vi "LaunchEditor.vi"(8 "error in (no error)":errorcluster {"code" format="Error %.0f"}, 10 "Editor Events":T1, 11 "Parser Settings In":refnum<class "Parser Settings.lvclass">) -> (0 "error out":errorcluster {"code" format="Error %.0f"}, 2 "VI Refnum":refnum<vi>, 3 "Parser Settings Out":refnum<class "Parser Settings.lvclass">)   [LabVIEW 2023, in "VIDoc Parsing.lvlib" / "Parser Settings.lvclass"]
uses:
  Parser Settings.lvclass
  Editors/VIDoc Editor/Editor Events Cluster.ctl
  Editor.vi
  Parser Settings.lvclass/Parser Settings.ctl
  Editors/VIDoc Editor/VIDocEditor.lvclass
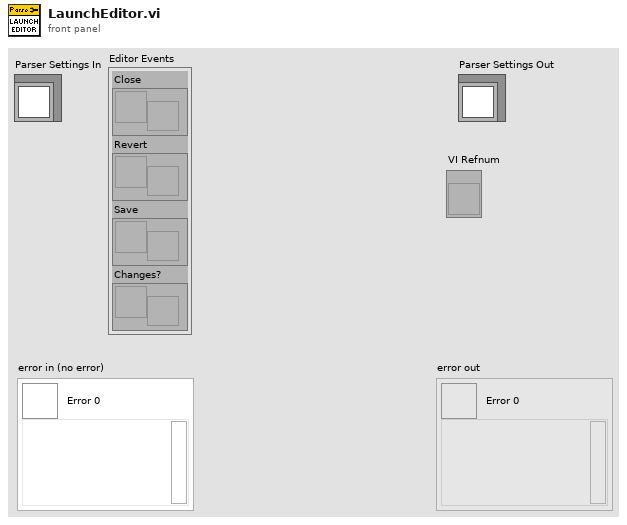
[diagram p1: front panel]
types:
  T1 = typedef "VIDocEditor.lvclass/Editor Events Cluster.ctl" = cluster{"Close":refnum<user-event>, "Revert":refnum<user-event>, "Save":refnum<user-event>, "Changes?":refnum<user-event>}
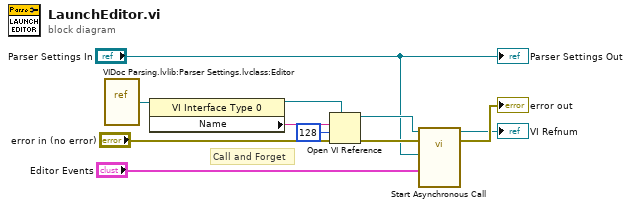
[diagram p0: block diagram]
diagram:
  # "Call and Forget"
  n1 = vi-ref "VIDoc Parsing.lvlib:Parser Settings.lvclass:Editor.vi"() -> (w11:refnum<vi>)
  n2 = property class="VI Interface Type 0"(reference=w11) -> (reference out=w10:refnum<vi>, "Name"=w9:string)  [unwired: 1 in, 1 out]
  n3 = Open VI Reference(type specifier VI Refnum (for type only)=w10, vi path=w9, options=128, error in (no error)="error in (no error)") -> (vi reference=w6:refnum<vi>, error out=w7:errorcluster)  [unwired: 2 in]
  n4 = call-by-ref "Start Asynchronous Call"(reference=w6, error in=w7, "Editor Events"="Editor Events", "Parser Settings In"="Parser Settings In") -> (reference out=→"VI Refnum":refnum<vi>, error out=→"error out":errorcluster)  [unwired: 9 in, 1 out]
  "Parser Settings Out" <- "Parser Settings In"
